vi "FT10_Unitherm Set Load.vi"(8 "error in (no error)":errorcluster, 9 "Load Impedance in":i32 max=6400 step=1, 11 "VISA Refnum in":refnum<visa-resource-name>) -> (0 "error out":errorcluster, 1 "Load Impedance out":i32 max=6400 step=1, 3 "VISA Refnum out":refnum<visa-resource-name>, 4 "Set Load Case":string="False Case")   [LabVIEW 2015]
doc: "Adjusts impedance on Unitherm to value received at Load Impedance control."
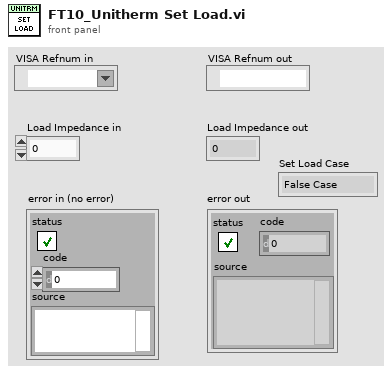
[diagram p1: front panel]
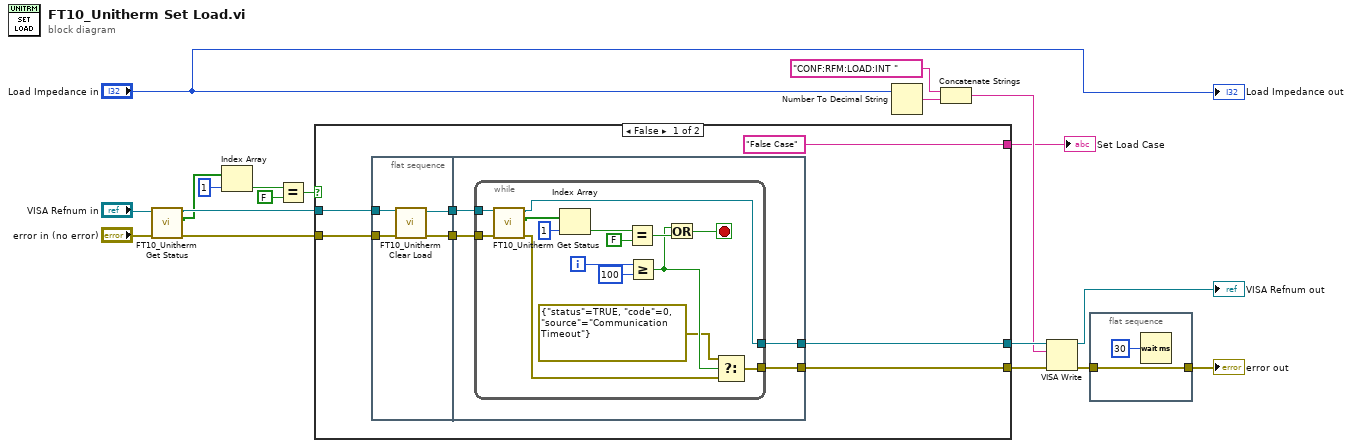
[diagram p0: block diagram]
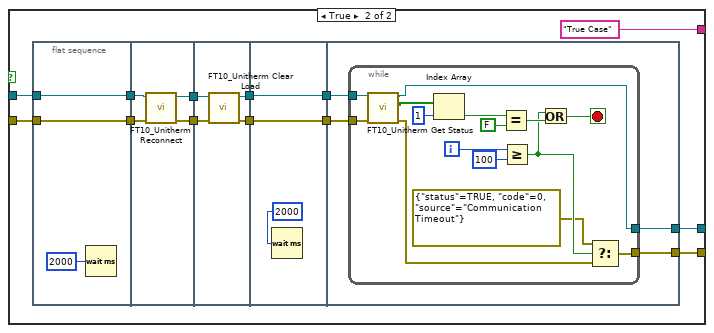
[diagram p2: hidden frame]
diagram:
  n1 = call "FT10_Unitherm Get Status.vi"("error in (no error)"="error in (no error)", "VISA Refnum in"="VISA Refnum in") -> ("error out"=w15:errorcluster, "Status"=w16:bool[], "VISA Refnum out"=w17:refnum<visa-resource-name>)  [unwired: 7 in]
  n2 = Index Array(array=w16, index=1) -> (element=w11:bool)
  n3 = Equal?(x=w11, y=FALSE) -> (x = y?=w10:bool)
  n4 = case shown="False" w10 {
    tunnel: w17 -> [w26 w60]
    tunnel: [w23 w55] -> w6
    tunnel: w15 -> [w25 w58]
    tunnel: [w24 w54] -> w7
    tunnel: ["False Case" "True Case"] -> w1
    frame False {
      n5 = flat-sequence {
        tunnel: w26 -> [w30]
        tunnel: w25 -> [w27]
        tunnel: [w28] -> w22
        tunnel: [w29] -> w21
        tunnel: w22 -> [w34]
        tunnel: w21 -> [w32]
        tunnel: [w33] -> w24
        tunnel: [w31] -> w23
        frame #0 {
          n6 = call "FT10_Unitherm Clear Load.vi"("error in (no error)"=w27, "VISA Refnum in"=w30) -> ("error out"=w28:errorcluster, "VISA Refnum out"=w29:refnum<visa-resource-name>)  [unwired: 7 in, 1 out]
        }
        frame #1 {
          n7 = while {
            tunnel: w34 -> [w36]
            tunnel: [w43] -> w33
            tunnel: w32 -> [w35]
            tunnel: [w39] -> w31
            i -> [w47]
            stop <- w49 stop-if-true
            n8 = call "FT10_Unitherm Get Status.vi"("error in (no error)"=w36, "VISA Refnum in"=w35) -> ("error out"=w37:errorcluster, "Status"=w38:bool[], "VISA Refnum out"=w39:refnum<visa-resource-name>)  [unwired: 7 in]
            n9 = Index Array(array=w38, index=1) -> (element=w41:bool)
            n10 = Equal?(x=w41, y=FALSE) -> (x = y?=w48:bool)
            n11 = Greater Or Equal?(x=w47, y=100 ("x")) -> (x >= y?=w45:bool)
            n12 = Or(x=w45, y=w48) -> (x .or. y?=w49:bool)
            n13 = Select(t=errorcluster {"status"=TRUE, "code"=0, "source"="Communication Timeout"} ("error out"), s=w45, f=w37) -> (s? t:f=w43:errorcluster)
          }
        }
      }
    }
    frame True {
      n14 = flat-sequence {
        tunnel: [w64] -> w61
        tunnel: w60 -> [w64]
        tunnel: [w63] -> w59
        tunnel: w58 -> [w63]
        tunnel: w61 -> [w69]
        tunnel: w59 -> [w68]
        tunnel: [w67] -> w57
        tunnel: [w66] -> w56
        tunnel: [w72] -> w53
        tunnel: [w73] -> w51
        tunnel: w57 -> [w71]
        tunnel: w56 -> [w70]
        tunnel: w53 -> [w76]
        tunnel: [w76] -> w52
        tunnel: w51 -> [w75]
        tunnel: [w75] -> w50
        tunnel: w52 -> [w80]
        tunnel: w50 -> [w78]
        tunnel: [w79] -> w54
        tunnel: [w77] -> w55
        frame #0 {
          n15 = Wait (ms)(milliseconds to wait=u32 2000) -> ()  [unwired: 1 out]
        }
        frame #1 {
          n16 = call "FT10_Unitherm Reconnect.vi"("error in (no error)"=w68, "VISA Refnum in"=w69) -> ("error out"=w66:errorcluster, "VISA Refnum out"=w67:refnum<visa-resource-name>)  [unwired: 8 in]
        }
        frame #2 {
          n17 = call "FT10_Unitherm Clear Load.vi"("error in (no error)"=w70, "VISA Refnum in"=w71) -> ("error out"=w72:errorcluster, "VISA Refnum out"=w73:refnum<visa-resource-name>)  [unwired: 7 in, 1 out]
        }
        frame #3 {
          n18 = Wait (ms)(milliseconds to wait=u32 2000) -> ()  [unwired: 1 out]
        }
        frame #4 {
          n19 = while {
            tunnel: w80 -> [w82]
            tunnel: [w89] -> w79
            tunnel: w78 -> [w81]
            tunnel: [w85] -> w77
            i -> [w93]
            stop <- w95 stop-if-true
            n20 = call "FT10_Unitherm Get Status.vi"("error in (no error)"=w82, "VISA Refnum in"=w81) -> ("error out"=w83:errorcluster, "Status"=w84:bool[], "VISA Refnum out"=w85:refnum<visa-resource-name>)  [unwired: 7 in]
            n21 = Index Array(array=w84, index=1) -> (element=w87:bool)
            n22 = Equal?(x=w87, y=FALSE) -> (x = y?=w94:bool)
            n23 = Greater Or Equal?(x=w93, y=100 ("x")) -> (x >= y?=w91:bool)
            n24 = Or(x=w91, y=w94) -> (x .or. y?=w95:bool)
            n25 = Select(t=errorcluster {"status"=TRUE, "code"=0, "source"="Communication Timeout"} ("error out"), s=w91, f=w83) -> (s? t:f=w89:errorcluster)
          }
        }
      }
    }
  }
  "Set Load Case" <- w1
  n26 = Number To Decimal String(number="Load Impedance in") -> (decimal integer string=w4:string)  [unwired: 1 in]
  n27 = Concatenate Strings("CONF:RFM:LOAD:INT " ("string"), w4) -> (w5:string)
  n28 = VISA Write(VISA resource name=w6, write buffer=w5, error in (no error)=w7) -> (VISA resource name out=→"VISA Refnum out":refnum<visa-resource-name>, error out=w13:errorcluster)  [unwired: 1 out]
  n29 = flat-sequence {
    tunnel: w13 -> [w96]
    tunnel: [w96] -> w14
    frame #0 {
      n30 = Wait (ms)(milliseconds to wait=u32 30) -> ()  [unwired: 1 out]
    }
  }
  "error out" <- w14
  "Load Impedance out" <- "Load Impedance in"
